vi "RW Noise Controller.vi"(11 "Expt State (in)":T2) -> (3 "Expt State":T2)   [LabVIEW 2020]
uses:
  Sub VIs/RWNoise Params.ctl
  epl-vi-lib/Utility VIs/Type Defs/Left-Right ring.ctl
  CFTS Main Panel SubVIs/CFTS-Experiment State.ctl
  CFTS Main Panel SubVIs/CFTS-Data Type Enum.ctl
panel:
  in  "Reject\nOverRide":bool
  in  "Rej Thresh µV":dbl=30.0
  out "Slide":dbl(slide) scale=0.0..1.0
  in  "Stim":T1={"Waveform"=enum."Pulses", "Freq (kHz)"=12.0, "Level (dB SPL)"=0.0, "Flo (kHz)"=8.0, "Fhi (kHz)"=16.0, "Ramp (ms)"=5.0, "Rep rate (/s)"=2.0, "Bursted?"=enum."Continuous", "Duration (ms)"=40.0, "Width (ms)"=1.0, "Rate (Hz)"=5.0}
  out "exit signal":bool
  out "Abort":bool
  out "User":string
  out "Run #":u16
  out "ID #":u16
  out "RW Noise (mV RMS)":dbl format="%#_3f"
  in  "Params":T3={"Sample rate (Hz)"=20000.0, "Sample duration (ms)"=128.0, "Grass gain"=10000.0, "Min Freq (Hz)"=673.0, "Max Freq (Hz)"=917.0, "Spectra to avg"=6, "Ear"=enum."Right"}
  out "Spectrum":waveform(dbl)(graph)
  out "Waveform":dbl[](graph)
  in  "START":bool
  in  "RETURN":bool
  in  "STOP":bool
  # "Spectrum"
  # "Stimulus"
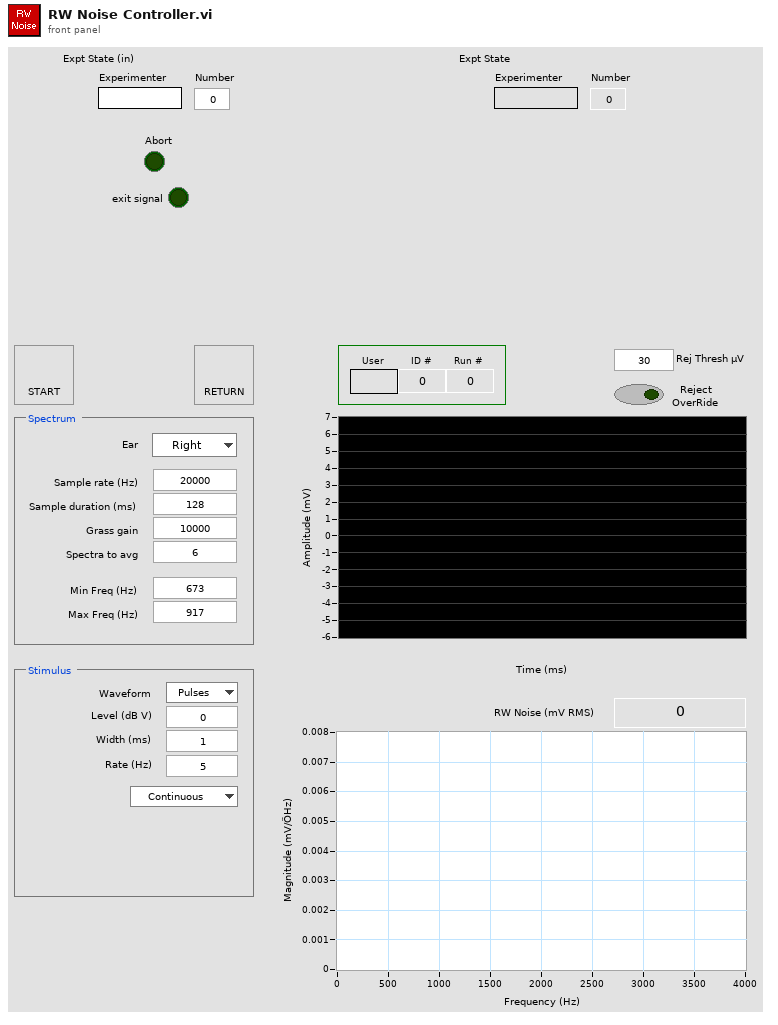
[diagram p1: front panel]
types:
  T1 = cluster{"Waveform":enum16{"OFF", "Tone", "Noise", "Pulses"}, "Freq (kHz)":dbl, "Level (dB SPL)":dbl, "Flo (kHz)":dbl, "Fhi (kHz)":dbl, "Ramp (ms)":dbl, "Rep rate (/s)":dbl, "Bursted?":enum16{"Continuous", "Bursted"}, "Duration (ms)":dbl, "Width (ms)":dbl, "Rate (Hz)":dbl}
  T2 = typedef "CFTS-Experiment State.ctl" = cluster{"Experimenter":string, "Number":u32, "Right":string, "Left":string, "Data Folder":path, "State File":path, "Version Info":string, "End Exposure Time":dbl, "Exposure Duration":string, "Run #":cluster{"CAP":i16, "ABR":i16, "DP":i16, "VsEP":i16, "MeasSeq":i16, "SubSeq":i16, "SFOAE":i16}}
  T3 = typedef "RWNoise Params.ctl" = cluster{"Sample rate (Hz)":dbl, "Sample duration (ms)":dbl, "Grass gain":dbl, "Min Freq (Hz)":dbl, "Max Freq (Hz)":dbl, "Spectra to avg":i32, "Ear":T4}
  T4 = typedef "Left-Right ring.ctl" = enum16{"Right", "Left"}
  T5 = cluster{"Shift":bool, "Ctrl":bool, "Alt":bool, "Cmd":bool, "Opt":bool}
  T6 = typedef "CFTS-Data Type Enum.ctl" = enum16{"CAP", "ABR", "DP", "VsEP", "MeasSeq", "SFOAE"}
  T7 = cluster{"Abort":refnum<vi>, "Waveform":refnum<vi>, "RW Noise (mV RMS)":refnum<vi>, "Spectrum":refnum<vi>, "Slide":refnum<vi>, "Rej Thresh µV":refnum<vi>, "Reject OverRide":refnum<vi>}
  T8 = typedef "RWNoise-Runtime Data.ctl" = cluster{"Stimulus":T9, "Fs (Hz)":dbl, "AO Npts":i32, "AO Channels":i32[], "Active":bool, "AINpts":i32, "WinPts":i32, "NUpdate":i32}
  T9 = typedef "Stimulus Channel (Full).xctl/Full Stimulus Channel Data.ctl" = cluster{"Waveform":T10, "Filter":T27, "Burst":T29, "Level":T30, "Name":string, "Advanced":T32, "SAM":T33}
  T10 = typedef "Waveform XCtl.xctl/Waveform Data.ctl" = cluster{"Type":T11, "Tone":T12, "Pulse Train":T13, "Noise":T16, "File":T17, "FMSweep":T18, "Chirp Train":T19, "Complex Tone":cluster{"Params":T21, "Data":T23}, "Moving Ripple":T24}
  T11 = typedef "Waveform Enum.ctl" = enum16{"OFF", "Tone", "Noise", "Pulse Train", "File", "FM Sweep", "Chirp Train", "Complex Tone", "FM Tone", "Moving Ripple"}
  T12 = typedef "Tone Params.ctl" = cluster{"Frequency (kHz)":dbl, "Last Freq":dbl, "Last Phase":dbl}
  T13 = typedef "Pulse Train Params.ctl" = cluster{"Pulse width (us)":dbl, "Pulse rate (Hz)":dbl, "Gap (ms)":dbl, "Polarity":T14, "PT State":T15, "Asynch":bool}
  T14 = typedef "Pulse Polarity.ctl" = enum16{"POS", "NEG", "POS-NEG", "NEG-POS"}
  T15 = typedef "PT-Continuous State.ctl" = cluster{"Template":dbl[], "Nperiod":i32, "Index":i32, "Pulse Rate (Hz)":dbl, "Phase (cycles)":dbl, "Noff":i32}
  T16 = typedef "Noise Params.ctl" = cluster{"InvFilt":bool, "Noise":dbl[], "CurPt":i32, "Aweight":bool, "Seed":i32, "afile":path}
  T17 = typedef "StimFile-Params.ctl" = cluster{"Filename":path, "Signal":dbl[], "Channel":i32, "stream":bool, "offset":i32, "nreps":i32, "loops":i32, "Randomize":bool, "order":i32[], "Seed":i32, "Tokens":i32}
  T18 = typedef "FM Sweep Params.ctl" = cluster{"Rate (oct/s)":dbl, "Fmin (Hz)":dbl, "Fmax (Hz)":dbl, "Ramp (ms)":dbl, "Linear":bool}
  T19 = typedef "Chirp Train.ctl" = cluster{"Params":T20, "Data":cluster{"WF":dbl[]}}
  T20 = typedef "Chirp Train Params.ctl" = cluster{"Fmin (kHz)":dbl, "Fmax (kHz)":dbl, "Compensate":bool, "Duration (ms)":dbl}
  T21 = typedef "CT-Params.ctl" = cluster{"F0 (Hz)":dbl, "Band":cluster{"Flow (Hz)":dbl, "Fhigh (Hz)":dbl}, "Phase":T22, "Min F0 (Hz)":dbl, "Max F0 (Hz)":dbl, "ContinRandPhase":bool, "Max peak factor":dbl, "Max mod depth":dbl, "MinHarmNum":i32, "MaxHarmNum":i32, "Level Mode":enum16{"per component", "overall rms"}, "% jitter":dbl}
  T22 = typedef "CT-Phase Enum.ctl" = enum16{"Cosine", "Random", "Alternating"}
  T23 = typedef "CT-Runtime Data.ctl" = cluster{"Ncomp":i32, "MinHarm":i32, "Phase":dbl[], "Amplitude":dbl[], "Npts/frame":i32, "Last F0":dbl, "Fmin":dbl, "Fmax":dbl, "Lslope":dbl, "randphase":bool, "overall rms":bool, "fmult":dbl[], "jittered":bool}
  T24 = typedef "Moving Ripple.ctl" = cluster{"Params":T25, "Data":T26}
  T25 = typedef "Moving Ripple.Params.ctl" = cluster{"Fmin":dbl, "Fmax":dbl, "Density":dbl, "Velocity":dbl, "Depth":dbl, "Phase":dbl, "Comp/oct":i32}
  T26 = typedef "Moving Ripple.Data.ctl" = cluster{"Freq":dbl[], "A":dbl[], "phase":dbl[], "Phase":dbl}
  T27 = typedef "Advanced Filter XCtl.xctl/Filter Data.ctl" = cluster{"Type":enum16{"Lowpass", "Highpass", "Bandpass", "Bandstop", "OFF"}, "CF (kHz)":dbl, "BW (kHz)":dbl, "Cascade":bool, "Quadrature":bool, "Scale Factor":dbl, "Stages":cluster{"IIR Filter":cluster{"filter structure":enum32{"IIR 2nd Order", "IIR 4th Order"}, "Reverse Coefficients":dbl[], "Forward Coefficients":dbl[]}, "State":dbl[]}[], "Class":enum16{"Elliptic", "Butterworth"}, "Order":i32, "BWUnits":T28}
  T28 = typedef "Filter-Bandwidth Units.ctl" = enum16{"Linear", "Octaves", "Min-Max"}
  T29 = typedef "Burst Control.xctl/Burst Data.ctl" = cluster{"Active":bool, "Delay (ms)":dbl, "Duration (ms)":dbl, "Ramp (ms)":dbl, "Rate (Hz)":dbl, "Trepeat (ms)":dbl, "Repeat":bool}
  T30 = typedef "Level XCtl.xctl/Level Data.ctl" = cluster{"Level":dbl, "Units":T31, "Max":dbl, "Multiplier":dbl, "Cal File":path, "Cal":cluster{"Freq (Hz)":dbl[], "Mag (dB SPL)":dbl[], "Phase (deg)":dbl[]}}
  T31 = typedef "Level Units.ctl" = enum16{"dB atten", "dB SPL", "dB re 1 Vrms", "dB V/Hz½", "mW", "dB HL", "Volts", "dB mW"}
  T32 = typedef "Advanced Stimulus Options.xctl/Advanced Stimulus Options.ctl" = cluster{"Rep Mask":string, "AltPol":bool, "Var":string, "Expr":string, "Persist":bool}
  T33 = typedef "SAM Params.ctl" = cluster{"Active":bool, "Frequency (Hz)":dbl, "Depth":dbl, "Init Phase (cycles)":dbl, "phase (degrees)":dbl, "Asynch":bool}
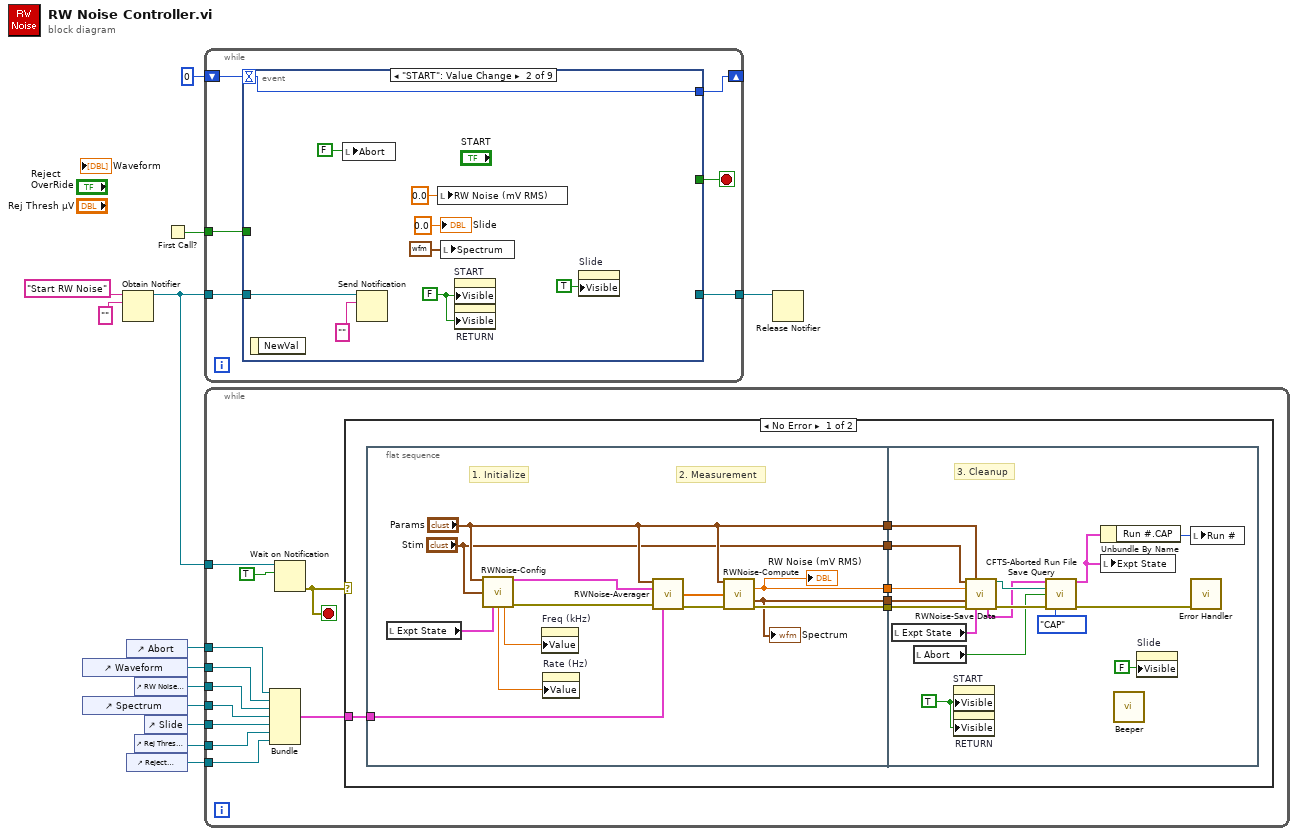
[diagram p0: block diagram]
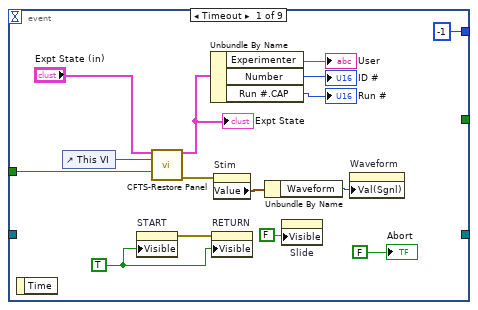
[diagram p3: hidden frame]
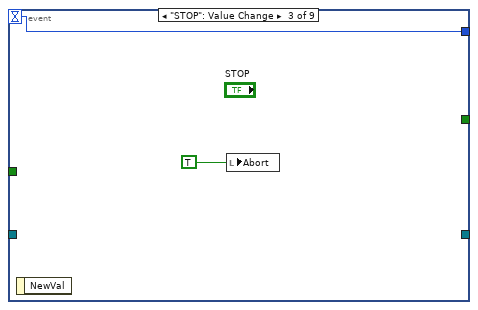
[diagram p4: hidden frame]
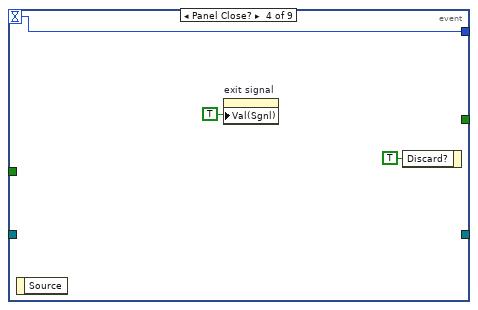
[diagram p5: hidden frame]
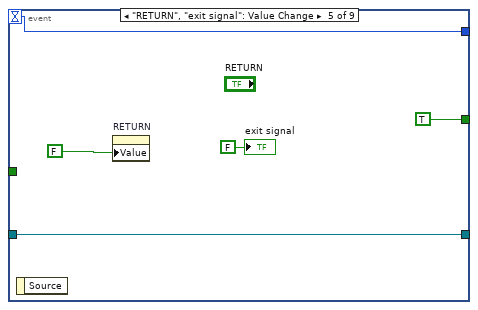
[diagram p6: hidden frame]
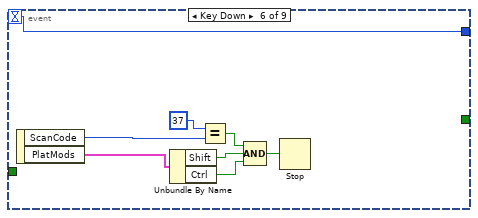
[diagram p7: hidden frame]
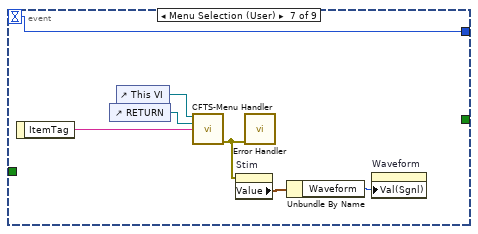
[diagram p8: hidden frame]
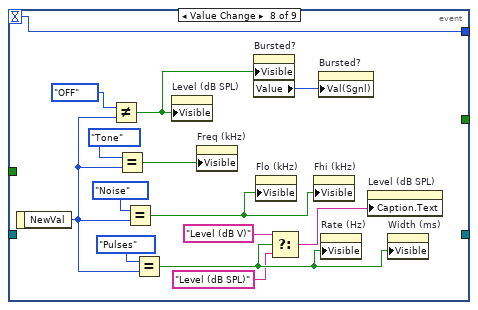
[diagram p9: hidden frame]
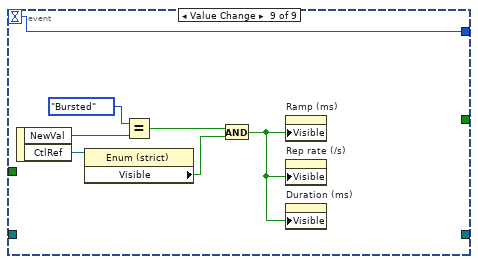
[diagram p10: hidden frame]
diagram:
  n1 = control-ref of="Waveform"() -> (w6:refnum<vi>)
  n2 = control-ref of="Spectrum"() -> (w4:refnum<vi>)
  n3 = Obtain Notifier(name (unnamed)="Start RW Noise", notification data type="") -> (notifier out=w13:refnum<notifier>)  [unwired: 2 in, 2 out]
  n4 = control-ref of="Abort"() -> (w7:refnum<vi>)
  n5 = control-ref of="Reject OverRide"() -> (w1:refnum<vi>)
  n6 = control-ref of="RW Noise (mV RMS)"() -> (w5:refnum<vi>)
  n7 = control-ref of="Rej Thresh µV"() -> (w2:refnum<vi>)
  n8 = control-ref of="Slide"() -> (w3:refnum<vi>)
  n9 = First Call?() -> (First Call?: T/F=w8:bool)
  n10 = while {
    tunnel: w13 -> [w19]
    tunnel: [w17] -> w12
    shift-right: [w15] -> _
    shift-left: 0 -> [w16]
    tunnel: w8 -> [w14]
    stop <- w18 stop-if-true
    n11 = event shown="[1] \"START\": Value Change" {
      selector: _ -> [_ _ _ _ _ _ _ _ _]
      dyn-events: _ -> [_ _ _ _ _ _ _ _ _]
      timeout: w16 -> [_ w41 w45 w48 w51 w54 w68 w82 w89]
      tunnel: w19 -> [_ w42 _ _ w52 _ _ _ _]
      tunnel: [_ _ _ _ TRUE _ _ _ _] -> w18
      tunnel: [_ _ _ _ w52 _ _ _ _] -> w17
      tunnel: [-1 w41 w45 w48 w51 w54 w68 w82 w89] -> w15
      tunnel: w14 -> [w25 _ _ _ _ _ _ _ _]
      event Timeout {
        w30 = TRUE ("Visible")
        n12 = event-data() -> ()  [unwired: 1 in, 1 out]
        n13 = control-ref of="This VI"() -> (w24:refnum<vi>)
        n14 = property on="START" class="Bool"("Visible"=w30) -> (error out=w29:errorcluster)  [unwired: 2 in, 1 out]
        n15 = call "CFTS-Restore Panel.vi"("State (in)"="Expt State (in)", "VI refnum"=w24, "Restore?"=w25) -> ("State"=w26:T2, "error out"=w22:errorcluster)  [unwired: 11 in]
        "Expt State" <- w26
        n16 = Unbundle By Name(w26) -> ("Experimenter"=→"User":string, "Number"=→"ID #":u32, "Run #.CAP"=→"Run #":i16)
        n17 = property on="RETURN" class="Bool (strict)"(error in=w29, "Visible"=w30) -> ()  [unwired: 1 in, 2 out]
        n18 = property on="Stim" class="Clust (strict)"(error in=w22) -> ("Value"=w21:T1)  [unwired: 1 in, 2 out]
        n19 = Unbundle By Name(w21) -> ("Waveform"=w23:enum16{"OFF", "Tone", "Noise", "Pulses"})
        n20 = property on="Slide" class="Slide (strict)"("Visible"=FALSE) -> ()  [unwired: 2 in, 2 out]
        n21 = property on="Waveform" class="Enum (strict)"("Val(Sgnl)"=w23) -> ()  [unwired: 2 in, 2 out]
        "Abort" <- FALSE ("Abort")
      }
      event "START": Value Change {
        w36 = FALSE ("Visible")
        n22 = event-data() -> ()  [unwired: 1 in, 1 out]
        n23 = local write "Abort"(FALSE ("Global Abort")) -> ()
        n24 = Send Notification(notification="", notifier=w42) -> ()  [unwired: 1 in, 2 out]
        n25 = local write "RW Noise (mV RMS)"(0.0 ("RW Noise (mV RMS)")) -> ()
        n26 = local write "Spectrum"(waveform(dbl) {"t0"=timestamp(0 s since 1904-01-01), "dt"=1.0, "Y"=[]} ("Spectrum")) -> ()
        n27 = property on="START" class="Bool"("Visible"=w36) -> ()  [unwired: 2 in, 2 out]
        n28 = property on="RETURN" class="Bool (strict)"("Visible"=w36) -> ()  [unwired: 2 in, 2 out]
        n29 = property on="Slide" class="Slide (strict)"("Visible"=TRUE) -> ()  [unwired: 2 in, 2 out]
        "Slide" <- 0.0 ("Slide")
      }
      event "STOP": Value Change {
        n30 = event-data() -> ()  [unwired: 1 in, 1 out]
        n31 = local write "Abort"(TRUE ("Global Abort")) -> ()
      }
      event Panel Close? {
        n32 = event-data() -> ()  [unwired: 1 in, 1 out]
        n33 = property on="exit signal" class="Bool (strict)"("Val(Sgnl)"=TRUE ("Value (Signaling)")) -> ()  [unwired: 2 in, 2 out]
        n34 = event-data("Discard?"=TRUE) -> ()  [unwired: 1 in, 1 out]
      }
      event "RETURN", "exit signal": Value Change {
        n35 = event-data() -> ()  [unwired: 1 in, 1 out]
        n36 = property on="RETURN" class="Bool (strict)"("Value"=FALSE) -> ()  [unwired: 2 in, 2 out]
        "exit signal" <- FALSE ("exit signal")
      }
      event Key Down {
        n37 = event-data() -> ("ScanCode"=w56:i16, "PlatMods"=w55:T5)  [unwired: 1 in]
        n38 = Unbundle By Name(w55) -> ("Shift"=w59:bool, "Ctrl"=w58:bool)
        n39 = Equal?(x=i16 37 ("y"), y=w56) -> (x = y?=w60:bool)
        n40 = Compound Arithmetic op=AND(w60, w59, w58) -> (w57:bool)
        n41 = Stop(stop? (T)=w57) -> ()
      }
      event Menu Selection (User) {
        n42 = event-data() -> ("ItemTag"=w65:string)  [unwired: 1 in]
        n43 = control-ref of="RETURN"() -> (w67:refnum<vi>)
        n44 = control-ref of="This VI"() -> (w66:refnum<vi>)
        n45 = call "CFTS-Menu Handler.vi"("VI Refnum"=w66, "Return Refnum"=w67, "ItemTag"=w65) -> ("error out"=w62:errorcluster)  [unwired: 11 in, 1 out]
        n46 = property on="Stim" class="Clust (strict)"(error in=w62) -> ("Value"=w63:T1)  [unwired: 1 in, 2 out]
        n47 = call "Error Handler.vi"("error in (no error)"=w62) -> ()  [unwired: 13 in, 2 out]
        n48 = Unbundle By Name(w63) -> ("Waveform"=w64:enum16{"OFF", "Tone", "Noise", "Pulses"})
        n49 = property on="Waveform" class="Enum (strict)"("Val(Sgnl)"=w64) -> ()  [unwired: 2 in, 2 out]
      }
      event "Stim.Waveform": Value Change {
        n50 = event-data() -> ("NewVal"=w74:enum16{"OFF", "Tone", "Noise", "Pulses"})  [unwired: 1 in]
        n51 = Not Equal?(x=enum16{"OFF", "Tone", "Noise"}."OFF" ("y"), y=w74) -> (x != y?=w78:bool)
        n52 = Equal?(x=enum16{"OFF", "Tone", "Noise"}."Tone" ("y"), y=w74) -> (x = y?=w76:bool)
        n53 = Equal?(x=enum16{"OFF", "Tone", "Noise"}."Noise" ("y"), y=w74) -> (x = y?=w75:bool)
        n54 = Equal?(x=enum16{"OFF", "Tone", "Noise", "Pulses"}."Pulses", y=w74) -> (x = y?=w72:bool)
        n55 = property on="Level (dB SPL)" class="DigNum (strict)"("Visible"=w78) -> ()  [unwired: 2 in, 2 out]
        n56 = property on="Freq (kHz)" class="DigNum (strict)"("Visible"=w76) -> ()  [unwired: 2 in, 2 out]
        n57 = property on="Bursted?" class="Enum (strict)"("Visible"=w78) -> ("Value"=w77:enum16{"Continuous", "Bursted"})  [unwired: 2 in, 2 out]
        n58 = property on="Flo (kHz)" class="DigNum (strict)"("Visible"=w75) -> ()  [unwired: 2 in, 2 out]
        n59 = Select(t="Level (dB V)", s=w72, f="Level (dB SPL)") -> (s? t:f=w70:string)
        n60 = property on="Fhi (kHz)" class="DigNum (strict)"("Visible"=w75) -> ()  [unwired: 2 in, 2 out]
        n61 = property on="Bursted?" class="Enum (strict)"("Val(Sgnl)"=w77) -> ()  [unwired: 2 in, 2 out]
        n62 = property on="Rate (Hz)" class="DigNum (strict)"("Visible"=w72) -> ()  [unwired: 2 in, 2 out]
        n63 = property on="Level (dB SPL)" class="DigNum (strict)"("Caption.Text"=w70) -> ()  [unwired: 2 in, 2 out]
        n64 = property on="Width (ms)" class="DigNum (strict)"("Visible"=w72) -> ()  [unwired: 2 in, 2 out]
      }
      event "Stim.Bursted?": Value Change {
        n65 = event-data() -> ("NewVal"=w87:enum16{"Continuous", "Bursted"}, "CtlRef"=w88:refnum<vi>)  [unwired: 1 in]
        n66 = property class="Enum (strict)"(reference=w88) -> ("Visible"=w84:bool)  [unwired: 1 in, 2 out]
        n67 = Equal?(x=enum16{"Continuous", "Bursted"}."Bursted", y=w87) -> (x = y?=w85:bool)
        n68 = And(x=w85, y=w84) -> (x .and. y?=w83:bool)
        n69 = property on="Ramp (ms)" class="DigNum (strict)"("Visible"=w83) -> ()  [unwired: 2 in, 2 out]
        n70 = property on="Rep rate (/s)" class="DigNum (strict)"("Visible"=w83) -> ()  [unwired: 2 in, 2 out]
        n71 = property on="Duration (ms)" class="DigNum (strict)"("Visible"=w83) -> ()  [unwired: 2 in, 2 out]
      }
    }
  }
  n72 = while {
    tunnel: w13 -> [w99]
    tunnel: w7 -> [w97]
    tunnel: w6 -> [w96]
    tunnel: w5 -> [w95]
    tunnel: w4 -> [w94]
    tunnel: w3 -> [w93]
    tunnel: w2 -> [w91]
    tunnel: w1 -> [w90]
    stop <- w98 stop-if-true
    n73 = Bundle("Abort"=w97, "Waveform"=w96, "RW Noise (mV RMS)"=w95, "Spectrum"=w94, "Slide"=w93, "Rej Thresh µV"=w91, "Reject OverRide"=w90) -> (w92:T7)  [unwired: 1 in]
    n74 = Wait on Notification(notifier=w99, ignore previous (F)=TRUE) -> (error out=w98:errorcluster)  [unwired: 2 in, 3 out]
    n75 = case shown="No Error" w98 {
      tunnel: w92 -> [w101 _]
      frame No Error {
        n76 = flat-sequence {
          tunnel: [w116] -> w106
          tunnel: ["Params"] -> w105
          tunnel: [w114] -> w104
          tunnel: [w115] -> w103
          tunnel: ["Stim"] -> w102
          tunnel: w101 -> [w110]
          tunnel: w106 -> [w135]
          tunnel: w105 -> [w122]
          tunnel: w104 -> [w132]
          tunnel: w103 -> [w131]
          tunnel: w102 -> [w121]
          frame #0 {
            # "1. Initialize"
            # "2. Measurement"
            n77 = local read "Expt State"() -> (w109:T2)
            n78 = call "RWNoise-Config.vi"("RW Noise Params"="Params", "RWN Stim"="Stim", "Expt State"=w109) -> ("Runtime"=w112:T8, "Coerced pulse rate (Hz)"=w107:dbl, "Freq (kHz)"=w108:dbl, "error out"=w119:errorcluster)  [unwired: 9 in]
            n79 = property on="Freq (kHz)" class="DigNum (strict)"("Value"=w108) -> ()  [unwired: 2 in, 2 out]
            n80 = property on="Rate (Hz)" class="DigNum (strict)"("Value"=w107) -> ()  [unwired: 2 in, 2 out]
            n81 = call "RWNoise-Averager.vi"("RW Noise Params"="Params", "Runtime"=w112, "error in (no error)"=w119, "Refs"=w110) -> ("Spectrum (uV)"=w117:dbl[], "error out"=w118:errorcluster)  [unwired: 10 in]
            n82 = call "RWNoise-Compute.vi"("RW Noise Params"="Params", "Spectrum (uV)"=w117, "error in (no error)"=w118) -> ("RW Noise (uV)"=w114:dbl, "Spectrum (uV/sqrt(Hz))"=w115:waveform(dbl), "error out"=w116:errorcluster)  [unwired: 10 in]
            "Spectrum" <- w115
            "RW Noise (mV RMS)" <- w114
          }
          frame #1 {
            w133 = TRUE ("Visible")
            # "3. Cleanup"
            n83 = local read "Expt State"() -> (w130:T2)
            n84 = local read "Abort"() -> (w126:bool)
            n85 = property on="START" class="Bool"("Visible"=w133) -> ()  [unwired: 2 in, 2 out]
            n86 = property on="RETURN" class="Bool (strict)"("Visible"=w133) -> ()  [unwired: 2 in, 2 out]
            n87 = call "RWNoise-Save Data.vi"("RWN Stim"=w121, "RW Noise Params"=w122, "RW Noise (uV)"=w132, "Spectrum (dB)"=w131, "error in (no error)"=w135, "Expt State"=w130) -> ("path"=w128:path, "Expt State out"=w127:T2, "error out"=w134:errorcluster)  [unwired: 7 in]
            n88 = call "CFTS-Aborted Run File Save Query.vi"("Expt State"=w127, "Path"=w128, "Aborted"=w126, "error in (no error)"=w134, "Data Type"=CFTS-Data_Type_Enum."CAP") -> ("Expt State out"=w124:T2, "error out"=w129:errorcluster)  [unwired: 8 in, 1 out]
            n89 = Unbundle By Name(w124) -> ("Run #.CAP"=w123:i16)
            n90 = local write "Expt State"(w124) -> ()
            n91 = call "Beeper.vi"() -> ()  [unwired: 5 in, 1 out]
            n92 = property on="Slide" class="Slide (strict)"("Visible"=FALSE) -> ()  [unwired: 2 in, 2 out]
            n93 = local write "Run #"(w123) -> ()
            n94 = call "Error Handler.vi"("error in (no error)"=w129) -> ()  [unwired: 13 in, 2 out]
          }
        }
      }
      frame Error {
      }
    }
  }
  n95 = Release Notifier(notifier=w12) -> ()  [unwired: 2 in, 3 out]
